vi "filter.insert.order.vi"(11 "filter.data.in":T1 {"get.state"."v"."Quantity" format="%.0x"; "get.state"."v"."OrderId" format="%.0x"; "mem.cmd"."ord.2"."v"."Quantity" format="%016x"; "mem.cmd"."ord.2"."v"."OrderId" format="%016x"; "mem.cmd"."ord.1"."v"."Quantity" format="%016x"; "mem.cmd"."ord.1"."v"."OrderId" format="%016x"; "mem.cmd"."ticker"."v"."Symbol" format="%016x"; "mem.cmd"."order.slot.value"."Quantity" format="%016x"; "mem.cmd"."order.slot.value"."OrderId" format="%016x"; "debug"."v"."slot.3" format="%.0x"; "debug"."v"."slot.2" format="%.0x"; "debug"."v"."slot.1" format="%.0x"; "debug"."v"."slot.0" format="%.0x"; "Scratch"."OrderId" format="%016x"; "hash.2"."data.in" format="%.0x"; "hash.2"."crc32.out" format="%.0x"; "hash.1"."data.in" format="%.0x"; "hash.1"."crc32.out" format="%.0x"}) -> (3 "filter.data.out":T1 {"get.state"."v"."Quantity" format="%.0x"; "get.state"."v"."OrderId" format="%.0x"; "mem.cmd"."ord.2"."v"."Quantity" format="%016x"; "mem.cmd"."ord.2"."v"."OrderId" format="%016x"; "mem.cmd"."ord.1"."v"."Quantity" format="%016x"; "mem.cmd"."ord.1"."v"."OrderId" format="%016x"; "mem.cmd"."ticker"."v"."Symbol" format="%016x"; "mem.cmd"."order.slot.value"."Quantity" format="%016x"; "mem.cmd"."order.slot.value"."OrderId" format="%016x"; "debug"."v"."slot.3" format="%.0x"; "debug"."v"."slot.2" format="%.0x"; "debug"."v"."slot.1" format="%.0x"; "debug"."v"."slot.0" format="%.0x"; "Scratch"."OrderId" format="%016x"; "hash.2"."data.in" format="%.0x"; "hash.2"."crc32.out" format="%.0x"; "hash.1"."data.in" format="%.0x"; "hash.1"."crc32.out" format="%.0x"})   [LabVIEW 2020]
uses:
  filter.states.ctl
  filter.debug.slot.ctl
  filter.debug.ctl
  order.slot.ctl
  ticker.slot.ctl
  ticker.slot.access.ctl
  order.slot.hm.ctl
  order.slot.access.ctl
  filter.memory.command.ctl
  Filter.lvclass
  filter.data.scratch.ctl
  filter.data.ctl
  Market.Data.Common/fpga/orderbook.command.ctl
  Market.Data.Common/fpga/fpganow.common.fpga.lvlib
  filter.state.slot.ctl
  filter.state.ctl
  Market.Data.Common/fpga/orderbook.command.type.ctl
  filter.hash.ctl
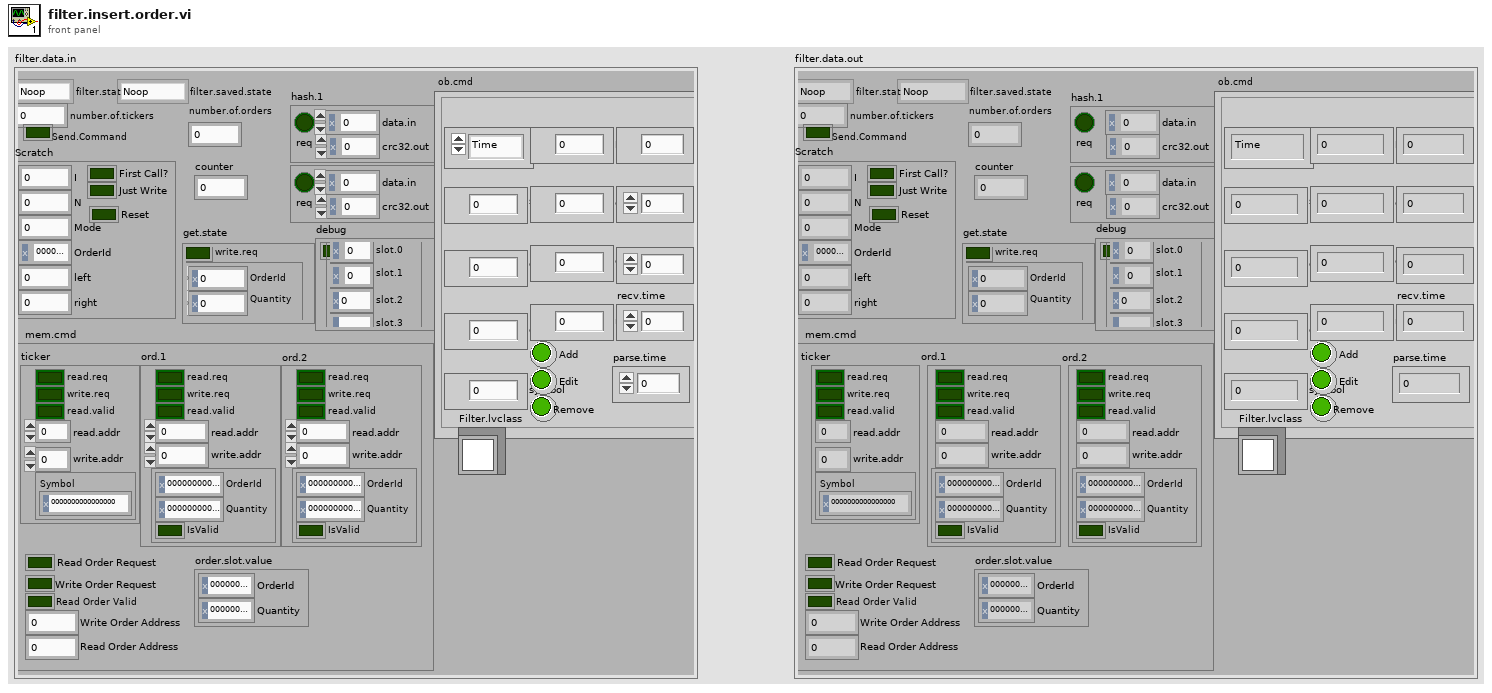
[diagram p1: front panel]
types:
  T1 = typedef "filter.data.ctl" = cluster{"filter.state":T2, "number.of.tickers":u32, "filter.saved.state":T2, "Send.Command":bool, "hash.1":T3, "hash.2":T3, "Scratch":T4, "debug":T5, "mem.cmd":T7, "get.state":T13, "ob.cmd":T15, "number.of.orders":u32, "Filter.lvclass":refnum<class "Filter.lvclass">, "counter":i16}
  T2 = typedef "filter.states.ctl" = enum16{"Noop", "Reset", "Debug", "Configuration", "Wait.for.Command", "Filter.Add", "Filter.Other", "Insert.Order", "Delete Order", "Get.State", "Get.Watchlist", "Get.Memory"}
  T3 = typedef "filter.hash.ctl" = cluster{"req":bool, "data.in":u64, "crc32.out":u32}
  T4 = typedef "filter.data.scratch.ctl" = cluster{"I":u32, "N":u32, "Mode":u32, "OrderId":u64, "First Call?":bool, "Just Write":bool, "left":u32, "right":u32, "Reset":bool}
  T5 = typedef "filter.debug.ctl" = cluster{"write":bool, "v":T6}
  T6 = typedef "filter.debug.slot.ctl" = cluster{"slot.0":u64, "slot.1":u64, "slot.2":u64, "slot.3":u64}
  T7 = typedef "filter.memory.command.ctl" = cluster{"Read Order Request":bool, "Write Order Request":bool, "Read Order Valid":bool, "Write Order Address":u32, "Read Order Address":u32, "order.slot.value":T8, "ticker":T9, "ord.1":T11, "ord.2":T11}
  T8 = typedef "order.slot.ctl" = cluster{"OrderId":u64, "Quantity":u64}
  T9 = typedef "ticker.slot.access.ctl" = cluster{"read.req":bool, "write.req":bool, "read.valid":bool, "read.addr":u32, "write.addr":u32, "v":T10}
  T10 = typedef "ticker.slot.ctl" = cluster{"Symbol":u64}
  T11 = typedef "order.slot.access.ctl" = cluster{"read.req":bool, "write.req":bool, "read.valid":bool, "read.addr":u32, "write.addr":u32, "v":T12}
  T12 = typedef "order.slot.hm.ctl" = cluster{"OrderId":u64, "Quantity":u64, "IsValid":bool}
  T13 = typedef "filter.state.ctl" = cluster{"write.req":bool, "v":T14}
  T14 = typedef "filter.state.slot.ctl" = cluster{"OrderId":u64, "Quantity":u64}
  T15 = typedef "fpganow.common.fpga.lvlib/orderbook.command.ctl" = cluster{"type":T16, "side":u8, "orderId ":u64, "quantity":u32, "symbol":u64, "price":u64, "executed.qty":u32, "canceled.qty":u32, "remaining.qty":u32, "seconds":u64, "nanoseconds":u64, "Add":bool, "Edit":bool, "Remove":bool, "seq no":u32, "recv.time":u64, "parse.time":u64}
  T16 = typedef "fpganow.common.fpga.lvlib/orderbook.command.type.ctl" = enum8{"Time", "AddOrder", "OrderExecuted", "OrderExecutedAtPrice", "ReduceSize", "ModifyOrder", "DeleteOrder", "Get.Everything", "Get.All.Orders", "Get.Top"}
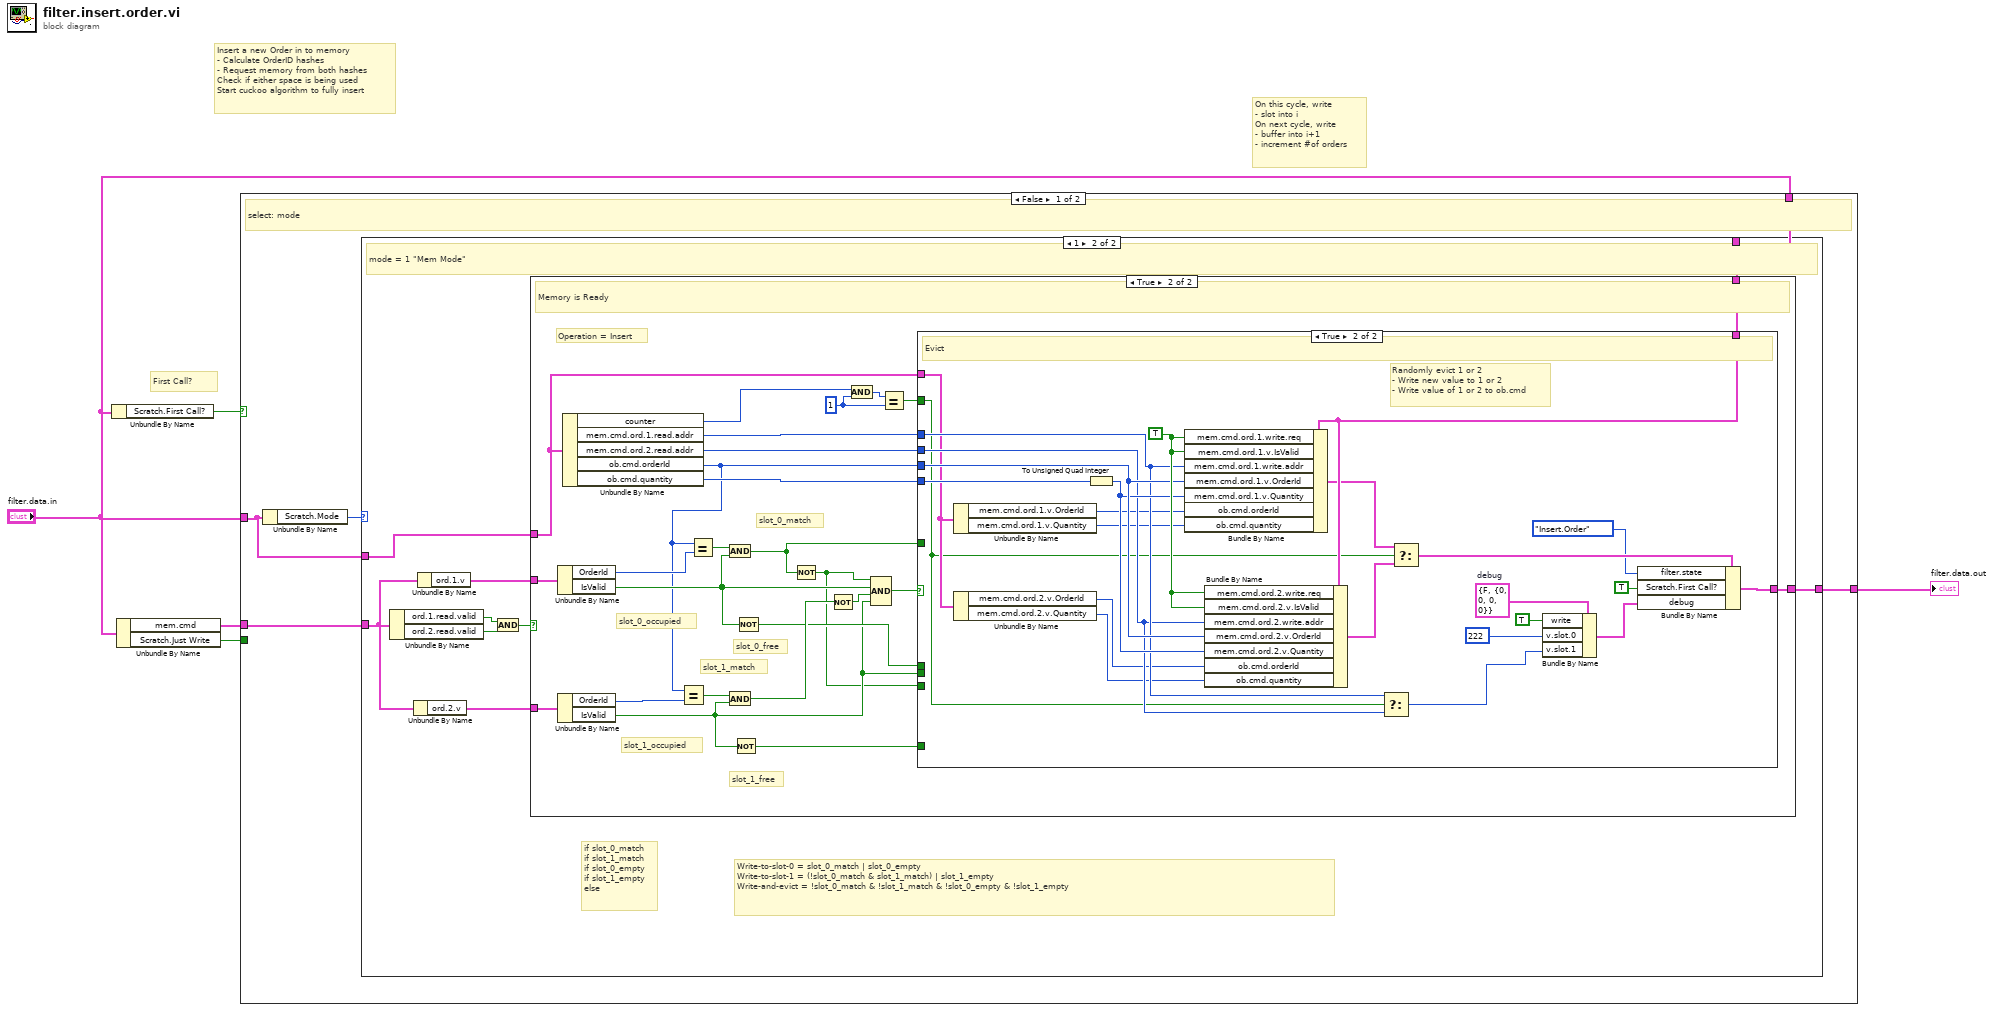
[diagram p0: block diagram]
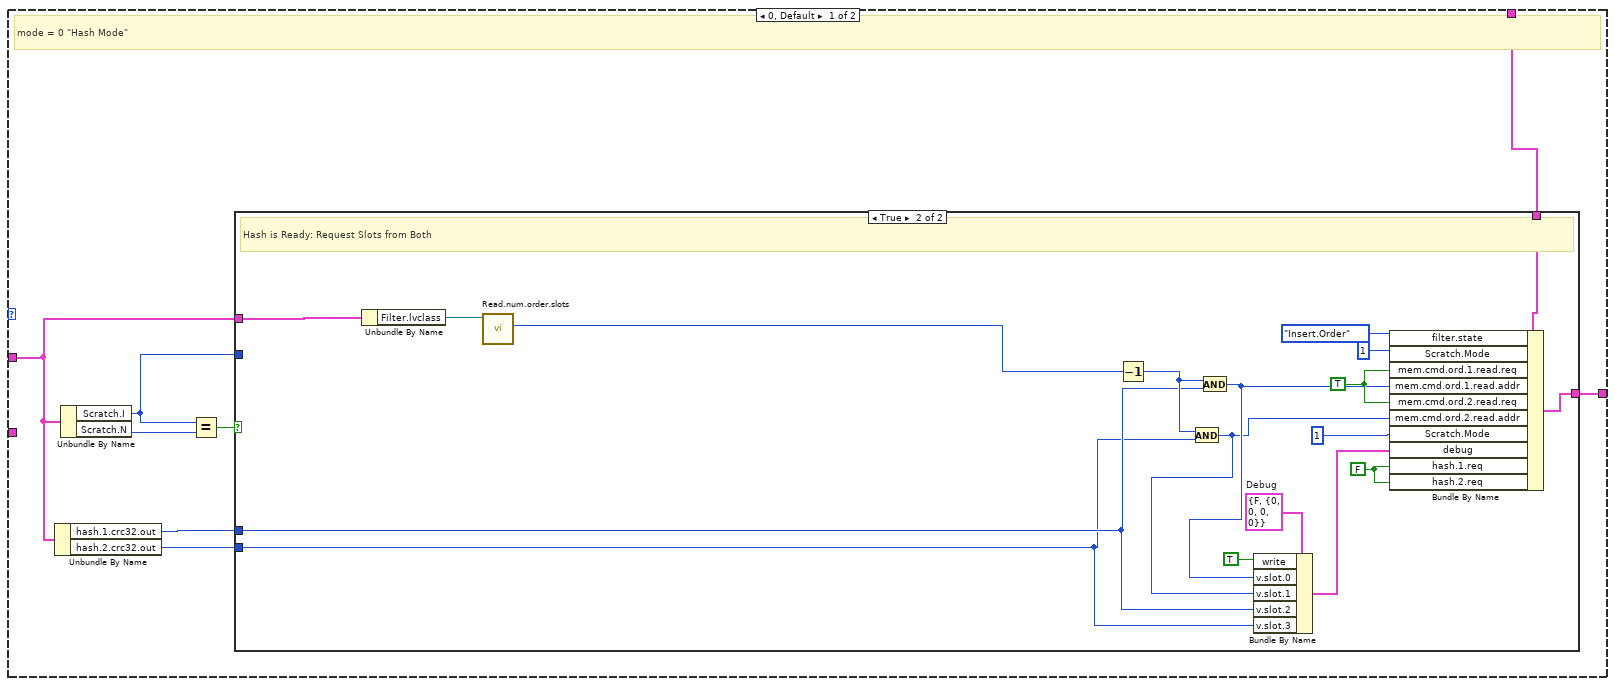
[diagram p2: hidden frame]
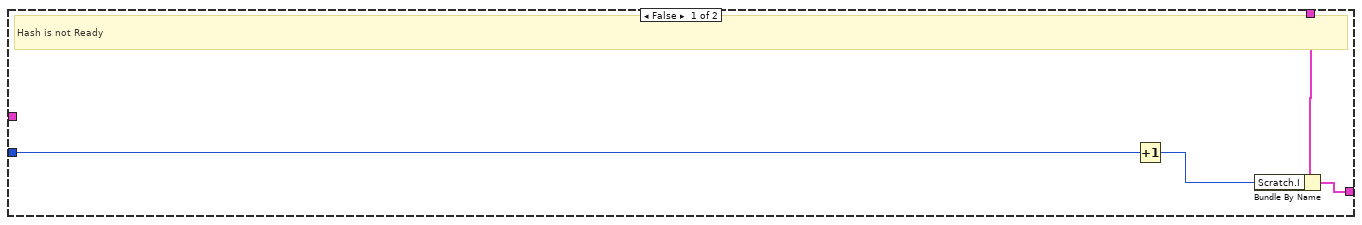
[diagram p3: hidden frame]
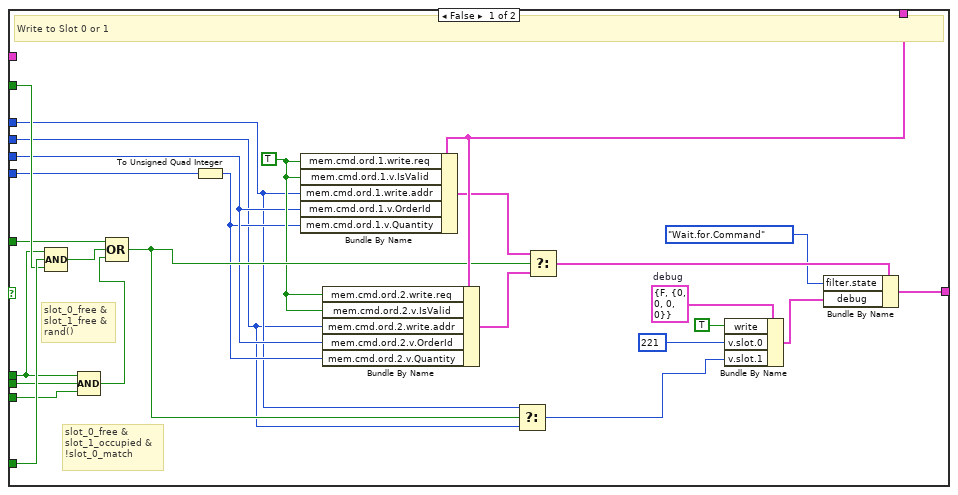
[diagram p5: hidden frame]
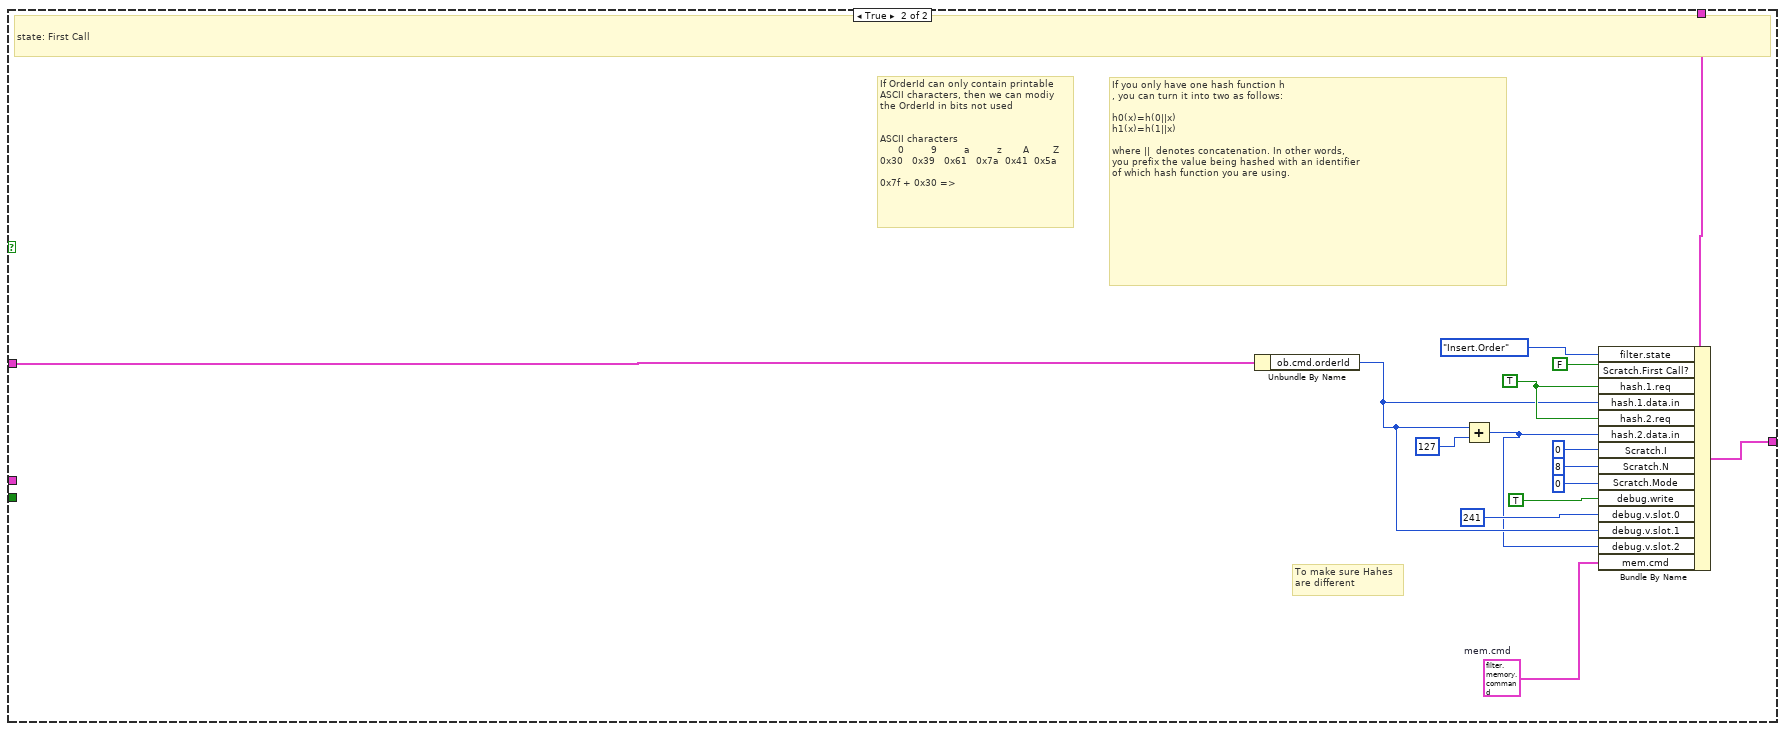
[diagram p6: hidden frame]
diagram:
  # "Insert a new Order in to memory\n- Calculate OrderID hashes\n- Request memory from both hashes\nCheck if either space is being used\nStart cuckoo algorithm to fully insert"
  # "On this cycle, write\n- slot into i\nOn next cycle, write\n- buffer into i+1\n- increment #of orders"
  # "First Call?"
  n1 = Unbundle By Name("filter.data.in") -> ("Scratch.First Call?"=w3:bool)
  n2 = Unbundle By Name("filter.data.in") -> ("mem.cmd"=w5:T7, "Scratch.Just Write"=w2:bool)
  n3 = case shown="False" w3 {
    tunnel: "filter.data.in" -> [w8 w141]
    tunnel: [w7 w138] -> w4
    tunnel: w5 -> [w6 _]
    tunnel: "filter.data.in" -> [w9 w139]
    tunnel: w2 -> [_ _]
    frame False {
      # "select: mode"
      n4 = Unbundle By Name(w9) -> ("Scratch.Mode"=w10:u32)
      n5 = case shown="1" w10 {
        tunnel: w9 -> [w11 w41]
        tunnel: w8 -> [w15 w46]
        tunnel: [w14 w45] -> w7
        tunnel: w6 -> [_ w44]
        frame 0, Default {
          # "mode = 0 \"Hash Mode\""
          n6 = Unbundle By Name(w11) -> ("hash.1.crc32.out"=w13:u32, "hash.2.crc32.out"=w12:u32)
          n7 = Unbundle By Name(w11) -> ("Scratch.I"=w16:u32, "Scratch.N"=w18:u32)
          n8 = Equal?(x=w16, y=w18) -> (x = y?=w17:bool)
          n9 = case shown="True" w17 {
            tunnel: w16 -> [w21 _]
            tunnel: w15 -> [w22 w40]
            tunnel: [w19 w39] -> w14
            tunnel: w13 -> [_ w25]
            tunnel: w12 -> [_ w24]
            tunnel: w11 -> [_ w28]
            frame False {
              # "Hash is not Ready"
              n10 = Increment(x=w21) -> (x+1=w20:u32)
              n11 = Bundle By Name(cluster=w22, "Scratch.I"=w20) -> (w19:T1)
            }
            frame True {
              w23 = FALSE ("hash.1.req")
              w33 = TRUE ("mem.cmd.ord.1.read.req")
              w37 = T5 {"write"=FALSE, "v"={"slot.0"=0, "slot.1"=0, "slot.2"=0, "slot.3"=0}}  # Debug
              # "Hash is Ready: Request Slots from Both"
              n12 = Unbundle By Name(w28) -> ("Filter.lvclass"=w27:refnum<class "Filter.lvclass">)
              n13 = call-dynamic "Read.num.order.slots.vi"("Filter in"=w27) -> ("num.order.slots"=w26:u32)  [unwired: 8 in, 2 out]
              n14 = Decrement(x=w26) -> (x-1=w34:u32)
              n15 = And(x=w34, y=w24) -> (x .and. y?=w29:u32)
              n16 = And(x=w34, y=w25) -> (x .and. y?=w30:u32)
              n17 = Bundle By Name(cluster=w37, "write"=TRUE ("Write.to.Debug"), "v.slot.0"=w30, "v.slot.1"=w29, "v.slot.2"=w25, "v.slot.3"=w24) -> (w31:T5)
              n18 = Bundle By Name(cluster=w40, "filter.state"=filter.states."Insert.Order", "Scratch.Mode"=u32 1, "mem.cmd.ord.1.read.req"=w33, "mem.cmd.ord.1.read.addr"=w30, "mem.cmd.ord.2.read.req"=w33, "mem.cmd.ord.2.read.addr"=w29, "Scratch.Mode"=u32 1, "debug"=w31, "hash.1.req"=w23, "hash.2.req"=w23) -> (w39:T1)
            }
          }
        }
        frame 1 {
          # "if slot_0_match\nif slot_1_match\nif slot_0_empty\nif slot_1_empty\nelse"
          # "Write-to-slot-0 = slot_0_match | slot_0_empty\nWrite-to-slot-1 = (!slot_0_match & slot_1_match) | slot_1_empty\nWrite-and-evict = !slot_0_match & !slot_1_match & !slot_0_empty & !slot_1_empty"
          # "mode = 1 \"Mem Mode\""
          n19 = Unbundle By Name(w44) -> ("ord.1.read.valid"=w48:bool, "ord.2.read.valid"=w49:bool)
          n20 = Unbundle By Name(w44) -> ("ord.2.v"=w42:T12)
          n21 = Unbundle By Name(w44) -> ("ord.1.v"=w43:T12)
          n22 = And(x=w48, y=w49) -> (x .and. y?=w47:bool)
          n23 = case shown="True" w47 {
            tunnel: w46 -> [w50 w70]
            tunnel: [w50 w69] -> w45
            tunnel: w43 -> [_ w76]
            tunnel: w42 -> [_ w75]
            tunnel: w41 -> [_ w51]
            frame False {
              # "Memory is not Ready"
            }
            frame True {
              w60 = i16 1 ("counter")
              # "slot_0_occupied"
              # "slot_0_free"
              # "slot_1_occupied"
              # "slot_1_free"
              # "slot_1_match"
              # "slot_0_match"
              # "Operation = Insert"
              # "Memory is Ready"
              n24 = Unbundle By Name(w76) -> ("OrderId"=w74:u64, "IsValid"=w66:bool)
              n25 = Unbundle By Name(w75) -> ("OrderId"=w73:u64, "IsValid"=w57:bool)
              n26 = Unbundle By Name(w51) -> ("counter"=w59:i16, "mem.cmd.ord.1.read.addr"=w55:u32, "mem.cmd.ord.2.read.addr"=w54:u32, "ob.cmd.orderId"=w52:u64, "ob.cmd.quantity"=w53:u32)
              n27 = Equal?(x=w52, y=w73) -> (x = y?=w71:bool)
              n28 = Equal?(x=w52, y=w74) -> (x = y?=w72:bool)
              n29 = And(x=w72, y=w66) -> (x .and. y?=w64:bool)
              n30 = And(x=w71, y=w57) -> (x .and. y?=w68:bool)
              n31 = Not(x=w57) -> (.not. x?=w62:bool)
              n32 = Not(x=w66) -> (.not. x?=w63:bool)
              n33 = Not(x=w64) -> (.not. x?=w56:bool)
              n34 = Not(x=w68) -> (.not. x?=w67:bool)
              n35 = And(x=w59, y=w60) -> (x .and. y?=w61:i16)
              n36 = Compound Arithmetic op=AND(w56, w66, w67, w57) -> (w65:bool)
              n37 = Equal?(x=w61, y=w60) -> (x = y?=w58:bool)
              n38 = case shown="True" w65 {
                tunnel: w70 -> [w102 w126]
                tunnel: [w98 w122] -> w69
                tunnel: w64 -> [w88 _]
                tunnel: w63 -> [w85 _]
                tunnel: w62 -> [w91 _]
                tunnel: w58 -> [w90 w105]
                tunnel: w57 -> [w84 _]
                tunnel: w56 -> [w83 _]
                tunnel: w55 -> [w78 w112]
                tunnel: w52 -> [w81 w115]
                tunnel: w54 -> [w77 w111]
                tunnel: w53 -> [w80 w114]
                tunnel: w51 -> [_ w110]
                frame False {
                  w82 = TRUE ("mem.cmd.ord.1.write.req")
                  w96 = T5 {"write"=FALSE, "v"={"slot.0"=0, "slot.1"=0, "slot.2"=0, "slot.3"=0}}  # debug
                  # "slot_0_free &\nslot_1_occupied &\n!slot_0_match"
                  # "slot_0_free & \nslot_1_free &\nrand()"
                  # "Write to Slot 0 or 1"
                  n39 = Compound Arithmetic op=AND(w85, w91, w90) -> (w89:bool)
                  n40 = Compound Arithmetic op=AND(w85, w84, w83) -> (w86:bool)
                  n41 = Compound Arithmetic op=OR(w88, w89, w86) -> (w87:bool)
                  n42 = To Unsigned Quad Integer(1:w80) -> (0:w79:u64)
                  n43 = Bundle By Name(cluster=w102, "mem.cmd.ord.1.write.req"=w82, "mem.cmd.ord.1.v.IsValid"=w82, "mem.cmd.ord.1.write.addr"=w78, "mem.cmd.ord.1.v.OrderId"=w81, "mem.cmd.ord.1.v.Quantity"=w79) -> (w101:T1)
                  n44 = Bundle By Name(cluster=w102, "mem.cmd.ord.2.write.req"=w82, "mem.cmd.ord.2.v.IsValid"=w82, "mem.cmd.ord.2.write.addr"=w77, "mem.cmd.ord.2.v.OrderId"=w81, "mem.cmd.ord.2.v.Quantity"=w79) -> (w100:T1)
                  n45 = Select(t=w78, s=w87, f=w77) -> (s? t:f=w92:u32)
                  n46 = Select(t=w101, s=w87, f=w100) -> (s? t:f=w99:T1)
                  n47 = Bundle By Name(cluster=w96, "write"=TRUE, "v.slot.0"=u64 221 ("v.Ticker"), "v.slot.1"=w92) -> (w95:T5)
                  n48 = Bundle By Name(cluster=w99, "filter.state"=filter.states."Wait.for.Command", "debug"=w95) -> (w98:T1)
                }
                frame True {
                  w116 = TRUE ("mem.cmd.ord.1.write.req")
                  w120 = T5 {"write"=FALSE, "v"={"slot.0"=0, "slot.1"=0, "slot.2"=0, "slot.3"=0}}  # debug
                  # "Randomly evict 1 or 2\n- Write new value to 1 or 2\n- Write value of 1 or 2 to ob.cmd"
                  # "Evict"
                  n49 = Unbundle By Name(w110) -> ("mem.cmd.ord.1.v.OrderId"=w109:u64, "mem.cmd.ord.1.v.Quantity"=w108:u64)
                  n50 = Unbundle By Name(w110) -> ("mem.cmd.ord.2.v.OrderId"=w106:u64, "mem.cmd.ord.2.v.Quantity"=w107:u64)
                  n51 = To Unsigned Quad Integer(1:w114) -> (0:w113:u64)
                  n52 = Bundle By Name(cluster=w126, "mem.cmd.ord.1.write.req"=w116, "mem.cmd.ord.1.v.IsValid"=w116, "mem.cmd.ord.1.write.addr"=w112, "mem.cmd.ord.1.v.OrderId"=w115, "mem.cmd.ord.1.v.Quantity"=w113, "ob.cmd.orderId"=w109, "ob.cmd.quantity"=w108) -> (w125:T1)
                  n53 = Bundle By Name(cluster=w126, "mem.cmd.ord.2.write.req"=w116, "mem.cmd.ord.2.v.IsValid"=w116, "mem.cmd.ord.2.write.addr"=w111, "mem.cmd.ord.2.v.OrderId"=w115, "mem.cmd.ord.2.v.Quantity"=w113, "ob.cmd.orderId"=w106, "ob.cmd.quantity"=w107) -> (w124:T1)
                  n54 = Select(t=w112, s=w105, f=w111) -> (s? t:f=w117:u32)
                  n55 = Select(t=w125, s=w105, f=w124) -> (s? t:f=w123:T1)
                  n56 = Bundle By Name(cluster=w120, "write"=TRUE, "v.slot.0"=u64 222 ("v.Ticker"), "v.slot.1"=w117) -> (w104:T5)
                  n57 = Bundle By Name(cluster=w123, "filter.state"=filter.states."Insert.Order", "Scratch.First Call?"=TRUE, "debug"=w104) -> (w122:T1)
                }
              }
            }
          }
        }
      }
    }
    frame True {
      w129 = T7 {"Read Order Request"=FALSE, "Write Order Request"=FALSE, "Read Order Valid"=FALSE, "Write Order Address"=0, "Read Order Address"=0, "order.slot.value"={"OrderId"=0, "Quantity"=0}, "ticker"={"read.req"=FALSE, "write.req"=FALSE, "read.valid"=FALSE, "read.addr"=0, "write.addr"=0, "v"={"Symbol"=0}}, "ord.1"={"read.req"=FALSE, "write.req"=FALSE, "read.valid"=FALSE, "read.addr"=0, "write.addr"=0, "v"={"OrderId"=0, "Quantity"=0, "IsValid"=FALSE}}, "ord.2"={"read.req"=FALSE, "write.req"=FALSE, "read.valid"=FALSE, "read.addr"=0, "write.addr"=0, "v"={"OrderId"=0, "Quantity"=0, "IsValid"=FALSE}}}  # mem.cmd
      w136 = TRUE ("hash.1.req")
      # "To make sure Hahes\nare different"
      # "If OrderId can only contain printable\nASCII characters, then we can modiy\nthe OrderId in bits not used\n\n\nASCII characters\n      0         9         a         z       A        Z\n0x30   0x39   0x61   0x7a  0x41  0x5a\n\n0x7f + 0x30 =>"
      # "If you only have one hash function h\n, you can turn it into two as follows:\n\nh0(x)=h(0||x)\nh1(x)=h(1||x)\n\nwhere ||  denotes concatenation. In other words,\nyou prefix the value being hashed with an identifier\nof which hash function you are using."
      # "state: First Call"
      n58 = Unbundle By Name(w139) -> ("ob.cmd.orderId"=w128:u64)
      n59 = Add(x=w128, y=u64 127) -> (x+y=w127:u64)
      n60 = Bundle By Name(cluster=w141, "filter.state"=filter.states."Insert.Order", "Scratch.First Call?"=FALSE, "hash.1.req"=w136, "hash.1.data.in"=w128, "hash.2.req"=w136, "hash.2.data.in"=w127, "Scratch.I"=u32 0, "Scratch.N"=u32 8, "Scratch.Mode"=u32 0, "debug.write"=TRUE ("Write.to.Debug"), "debug.v.slot.0"=u64 241 ("Debug.debug.slot.Ticker"), "debug.v.slot.1"=w128, "debug.v.slot.2"=w127, "mem.cmd"=w129) -> (w138:T1)
    }
  }
  "filter.data.out" <- w4
